vi "All Cal to CSV.vi"(8 "error in (no error)":errorcluster, 11 "Array":string[](array[string])) -> (0 "error out":errorcluster)   [LabVIEW 2018, in "Logging.lvlib"]
uses:
  Logging.lvlib
  <vilib>/Utility/file.llb/Write Delimited Spreadsheet (string).vi
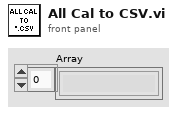
[diagram p1: front panel]
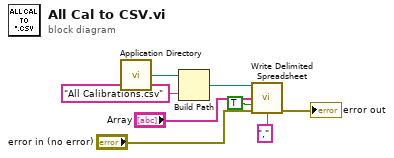
[diagram p0: block diagram]
diagram:
  n1 = call <vilib>:"Application Directory.vi"() -> ("Application Directory"=w1:path)
  n2 = Build Path(base path=w1, name or relative path="All Calibrations.csv") -> (appended path=w3:path)
  n3 = call-poly <vilib>:"Write Delimited Spreadsheet.vi"("file path (dialog if empty)"=w3, "1D data"="Array", "append to file? (new file:F)"=TRUE, "error in (no error)"="error in (no error)", "delimiter (\\t)"="," ("delimiter (\\t)")) -> ("error out"=→"error out":errorcluster)  [unwired: 9 in, 1 out]
